vi "DriverStationPushData.vi"   [LabVIEW 2018]
uses:
  d45ba836-02d8-4962-bfcd-028c5a01eed1.vi
  8d6ec62f-e14d-40c9-b57a-da8c82ab6d12.vi
  dsdata.vi
  constants.vi
  <vilib>/Rock Robotics/Network Tables/NT Write String Array.vi
  robotmodes.vi
  <vilib>/Rock Robotics/Network Tables/NT Write String.vi
types:
  T1 = typedef "WPI_DriverStationRobotMode2.ctl" = enum16{"Autonomous Disabled", "Autonomous Enabled", "Teleop Disabled", "Teleop Enabled", "Disconnected", "Finish", "Test Disabled", "Test Enabled", "Emergency Stopped"}
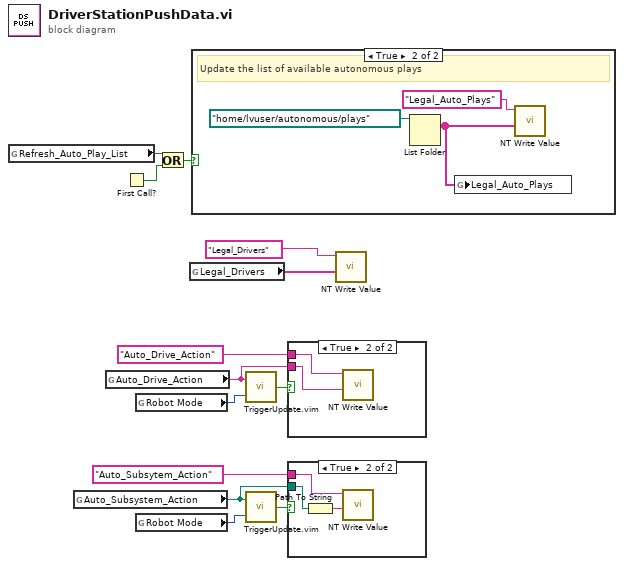
[diagram p0: block diagram]
diagram:
  n1 = global read "dsdata.vi" "Refresh_Auto_Play_List"() -> (w11:bool)
  n2 = global read "robotmodes.vi" "Auto_Subsystem_Action"() -> (w2:path)
  n3 = global read "robotmodes.vi" "Auto_Drive_Action"() -> (w6:string)
  n4 = First Call?() -> (First Call?: T/F=w10:bool)
  n5 = global read "dsdata.vi" "Robot Mode"() -> (w8:T1)
  n6 = global read "dsdata.vi" "Robot Mode"() -> (w4:T1)
  n7 = Or(x=w11, y=w10) -> (x .or. y?=w9:bool)
  n8 = global read "constants.vi" "Legal_Drivers"() -> (w13:string[])
  n9 = case shown="True" w9 {
    frame False {
    }
    frame True {
      # "Update the list of available autonomous plays"
      n10 = List Folder(path=path "/home/lvuser/autonomous/plays") -> (filenames=w14:string[])  [unwired: 3 in, 3 out]
      n11 = global write "constants.vi" "Legal_Auto_Plays"(w14) -> ()
      n12 = call-poly <vilib>:"NT Write Value.vi"("String Array"=w14, "Name"="Legal_Auto_Plays") -> ()  [unwired: 9 in, 1 out]
    }
  }
  n13 = call "TriggerUpdate.vim"("Robot Mode"=w8, "Trigger"=w6) -> ("Update"=w7:bool)
  n14 = call "TriggerUpdate.vim"("Robot Mode"=w4, "Trigger"=w2) -> ("Update"=w3:bool)
  n15 = case shown="True" w7 {
    tunnel: w6 -> [_ w18]
    tunnel: "Auto_Drive_Action" ("Name") -> [_ w17]
    frame False {
    }
    frame True {
      n16 = call-poly <vilib>:"NT Write Value.vi"("String"=w18, "Name"=w17) -> ()  [unwired: 9 in, 1 out]
    }
  }
  n17 = case shown="True" w3 {
    tunnel: w2 -> [_ w20]
    tunnel: "Auto_Subsytem_Action" ("Name") -> [_ w21]
    frame False {
    }
    frame True {
      n18 = Path To String(path=w20) -> (string=w19:string)
      n19 = call-poly <vilib>:"NT Write Value.vi"("String"=w19, "Name"=w21) -> ()  [unwired: 9 in, 1 out]
    }
  }
  n20 = call-poly <vilib>:"NT Write Value.vi"("String Array"=w13, "Name"="Legal_Drivers") -> ()  [unwired: 9 in, 1 out]
